vi "AlliGator Global 2-Exp + IRF Convolution Fit v2.vi"(0 "Decays":cluster{"t Array":dbl[], "Data Array":dbl[]}[](array[cluster]), 1 "Initial Parameters":dbl[](array[numeric])=[-1.0, 0.0, 0.5, 0.1, 0.5, 1.0], 2 "Optimal Offset Selection Criterion":T2, 5 "Global Fit Parameters Info":T11={"Fit Data"=variant(cluster{"t Array":dbl[], "IRF Array":dbl[]} {"t Array"=[], "IRF Array"=[]}), "Global Fit Parameter Information"={"Original Parameter Indices"=[], "# Global Parameters"=0, "# Plot Specific Parameters"=0, "Global Parameter? Array"=[]}, "# Points in Plots"=[]}, 9 "Fit Options":T14={"Show Fit Residuals"=TRUE, "Fit Model"=enum."1-Exponential", "Residual Type"=enum."Standard", "Max Decay Percentile"=0.0, "Min Decay Percentile"=0.0, "Show Full Decay"=TRUE, "Weights"=enum."Unweighted", "Fitting Method"=enum."Least Square", "Compute Parameter Uncertainties"=TRUE, "Periodic Boundaries"=TRUE, "Model Calculation"=enum."Simulation", "Period"=1.2500000000000001e-08, "Termination Criteria"={"Max Iterations"=1000, "Max Function Calls"=0, "Max Time"=1000.0, "Function Tolerance"=1e-06, "Parameter Tolerance"=1e-06, "Gradient Tolerance"=0.0, "Min Lambda"=1e-06, "Max Lambda"=1e-06, "Initial Tick Count"=0}, "Offset Resolution"=1.2500000000000001e-08, "Use Local IRF"=TRUE, "Fitting Algorithm"=enum."Levenberg-Marquardt", "Show Confidence Interval "=TRUE, "Confidence Level"=95.0} {"Confidence Level" min=0.0 max=100.0; "Offset Resolution" min=0.0; "Period" min=0.0; "Min Decay Percentile" min=0.0 max=1.0; "Max Decay Percentile" min=0.0 max=100.0}, 11 "error in (no error)":errorcluster, 12 "parameter bounds":T13, 13 "Termination Criteria":T3={"Max Iterations"=1000, "Max Function Calls"=10000, "Max Time"=1000.0, "Function Tolerance"=1e-06, "Parameter Tolerance"=1e-06, "Gradient Tolerance"=1e-06, "Min Lambda"=1e-06, "Max Lambda"=1e-06, "Initial Tick Count"=0}) -> (4 "Fit Plots Array":T1[](array[typedef]), 8 "Fit Output":T4={"best nonlinear fit"=[], "best fit parameters"=[], "R^2"=0.0, "RMSE"=0.0, "error out"={"status"=FALSE, "code"=0, "source"=""}, "Fitting Method"=enum."Least Square", "number of function calls"=0, "number of iterations"=0, "covariance"=[], "Chi 2"=0.0, "DOF"=0, "Fit Convergence Criterion"=enum."Continue", "Fitting Algorithm"=enum."Levenberg-Marquardt", "Weighted Fit"=enum."Unweighted", "Gradient"=0.0, "|Delta Chi 2|"=0.0, "|Delta Chi 2|/Chi 2"=0.0, "Max |Delta a| /|a|"=0.0, "Lambda"=-1.0, "RSS"=0.0, "AIC"=0.0, "BIC"=0.0, "Max number of function calls"=0, "Max number of iterations"=0, "IRF"={"X Array"=[], "Y Array"=[]}, "IRF Normalization Factor"=0.0, "Decay Normalization Factor"=0.0, "Number of offset fits"=0, "Weighted Chi2"=-1.0, "Unweighted Chi2"=-1.0}, 10 "Delta Best Fit Parameters":dbl[](array[numeric]), 15 "error out":errorcluster)   [LabVIEW 2021, in "AlliGator Global Decay Fit.lvlib"]
uses:
  AlliGator Global Decay Fit.lvlib
  Fits/IRF(X)PSED/Decay Fit Options v4.ctl
  Fits/Decay Convolution/Decay Model.ctl
  Fits/Residual Type.ctl
  Fits/IRF(X)PSED/Fit Weights Type v2.ctl
  Fits/Non-linear Fitting Method v2.ctl
  Fits/Fit Calculation Method.ctl
  Fits/Non-linear Fitting Algorithm.ctl
  Fits/Global Fits/Global Fit Data.ctl
  Fits/Global Fits/Global Fit Parameters Information.ctl
  Fits/Non-linear Fit Output v4.ctl
  Fits/Nonlinear Fit Method.ctl
  <vilib>/Analysis/Matrix/Datatypes/RealMatrix.ctl
  Fits/Convergence Criteria.ctl
  Graphs/XY Graph/XY Graph Plot Data.ctl
  Fits/My Fit Stopping Criteria.ctl
  Fits/Optimal Offset Selection Criterion.ctl
  Fits/Fit Plots.ctl
  Settings/AlliGator Settings List.ctl
  Fits/Decay Convolution/Fit Control Data.ctl
  Fits/Decay Convolution/Global LM model function and gradient (2-Exp + IRF) v2.vi
  Phasor/Phasor Abort Parallel Computation.vi
  Fits/Decay Convolution/Global LM model function and gradient (2-Exp, Convolved, Periodic).vi
  <vilib>/Utility/error.llb/Error Cluster From Error Code.vi
  <vilib>/ErrorRing/Error Ring.xnode
  Arrays/Arrays.lvlib
  Time/Time.lvlib
  Fits/Fits.lvlib
  Graphs/XY Graph/XY Graph Add-Ons.lvlib
  Settings/AlliGator Settings.lvlib
  Phasor/Phasor.lvlib
  Decay Fit/AlliGator Decay Fit.lvlib
  <vilib>/Analysis/Matrix/NI_Matrix.lvlib
panel:
  out "CPU (s)":dbl
  out "XY Graph":T19(graph)
  # "Offset\nBaseline\nA1\ntau1\nA2\ntau2"
  # "Offset\nBaseline\nA1\ntau 1\nA2\ntau 2"
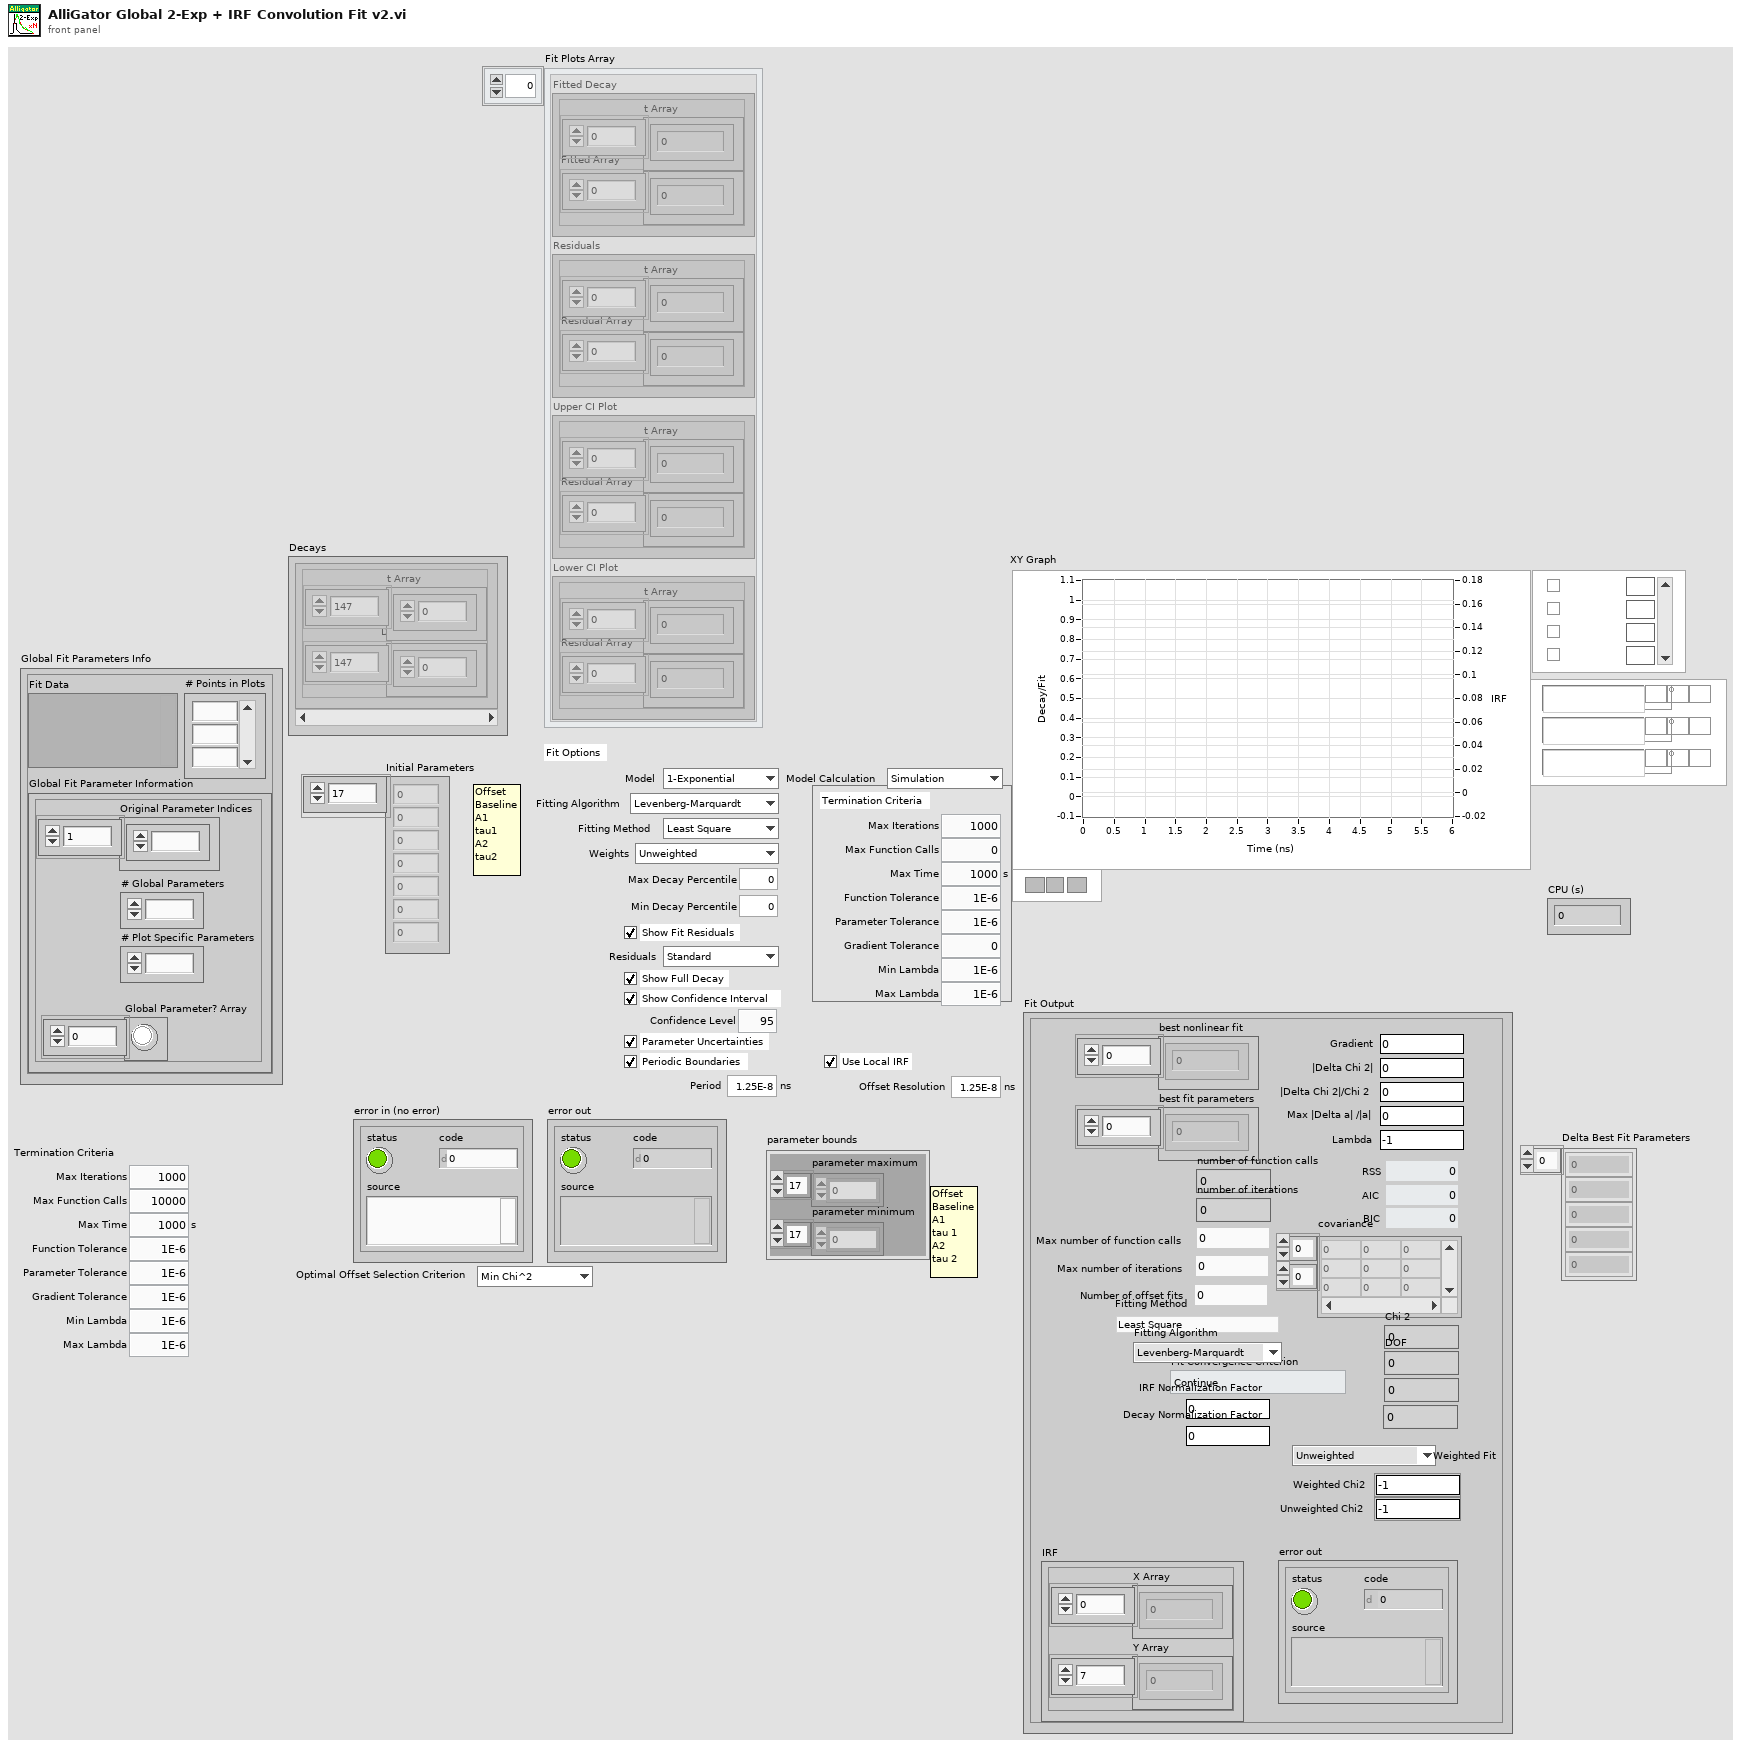
[diagram p1: front panel]
types:
  T1 = typedef "Fits.lvlib/Fit Plots.ctl" = cluster{"Fitted Decay":cluster{"t Array":dbl[], "Fitted Array":dbl[]}, "Residuals":cluster{"t Array":dbl[], "Residual Array":dbl[]}, "Upper CI Plot":cluster{"t Array":dbl[], "Residual Array":dbl[]}, "Lower CI Plot":cluster{"t Array":dbl[], "Residual Array":dbl[]}}
  T2 = typedef "Fits.lvlib/Optimal Offset Selection Criterion.ctl" = enum16{"Min Chi^2", "Max R^2"}
  T3 = typedef "Fits.lvlib/My Fit Stopping Criteria.ctl" = cluster{"Max Iterations":i32, "Max Function Calls":i32, "Max Time":dbl[unit], "Function Tolerance":dbl, "Parameter Tolerance":dbl, "Gradient Tolerance":dbl, "Min Lambda":dbl, "Max Lambda":dbl, "Initial Tick Count":u32}
  T4 = typedef "Fits.lvlib/Non-linear Fit Output v4.ctl" = cluster{"best nonlinear fit":dbl[], "best fit parameters":dbl[], "R^2":dbl, "RMSE":dbl, "error out":errorcluster, "Fitting Method":T5, "number of function calls":i32, "number of iterations":i32, "covariance":T6, "Chi 2":dbl, "DOF":i32, "Fit Convergence Criterion":T7, "Fitting Algorithm":T8, "Weighted Fit":T9, "Gradient":dbl, "|Delta Chi 2|":dbl, "|Delta Chi 2|/Chi 2":dbl, "Max |Delta a| /|a|":dbl, "Lambda":dbl, "RSS":dbl, "AIC":dbl, "BIC":dbl, "Max number of function calls":i32, "Max number of iterations":i32, "IRF":T10, "IRF Normalization Factor":dbl, "Decay Normalization Factor":dbl, "Number of offset fits":i32, "Weighted Chi2":dbl, "Unweighted Chi2":dbl}
  T5 = typedef "Fits.lvlib/Nonlinear Fit Method.ctl" = enum16{"Least Square", "Least Absolute Residual", "Bisquare", "MLE"}
  T6 = typedef "NI_Matrix.lvlib/RealMatrix.ctl" = dbl[][]
  T7 = typedef "Fits.lvlib/Convergence Criteria.ctl" = enum16{"Continue", "Tolerances Exceeded", "Max Time Exceeded", "Max Iterations Exceeded", "Max Function Evaluations Exceeded", "Scale Range Exceeded"}
  T8 = typedef "Fits.lvlib/Non-linear Fitting Algorithm.ctl" = enum16{"Levenberg-Marquardt", "Trust-Region Dogleg"}
  T9 = typedef "Fits.lvlib/Fit Weights Type v2.ctl" = enum16{"Unweighted", "1/Variance (Neyman)", "1/Variance (Pearson)", "Best of All"}
  T10 = typedef "XY Graph Add-Ons.lvlib/XY Graph Plot Data.ctl" = cluster{"X Array":dbl[], "Y Array":dbl[]}
  T11 = typedef "Fits.lvlib/Global Fit Data.ctl" = cluster{"Fit Data":variant, "Global Fit Parameter Information":T12, "# Points in Plots":i32[]}
  T12 = typedef "Fits.lvlib/Global Fit Parameters Information.ctl" = cluster{"Original Parameter Indices":i32[], "# Global Parameters":i32, "# Plot Specific Parameters":i32, "Global Parameter? Array":bool[]}
  T13 = cluster{"parameter minimum":dbl[], "parameter maximum":dbl[]}
  T14 = typedef "Fits.lvlib/Decay Fit Options v4.ctl" = cluster{"Show Fit Residuals":bool, "Fit Model":T15, "Residual Type":T16, "Max Decay Percentile":dbl, "Min Decay Percentile":dbl, "Show Full Decay":bool, "Weights":T9, "Fitting Method":T17, "Compute Parameter Uncertainties":bool, "Periodic Boundaries":bool, "Model Calculation":T18, "Period":dbl[unit], "Termination Criteria":cluster{"Max Iterations":i32, "Max Function Calls":i32, "Max Time":dbl[unit], "Function Tolerance":dbl, "Parameter Tolerance":dbl, "Gradient Tolerance":dbl, "Min Lambda":dbl, "Max Lambda":dbl, "Initial Tick Count":u32}, "Offset Resolution":dbl[unit], "Use Local IRF":bool, "Fitting Algorithm":T8, "Show Confidence Interval ":bool, "Confidence Level":dbl}
  T15 = typedef "Fits.lvlib/Decay Model.ctl" = enum16{"1-Exponential", "2-Exponentials"}
  T16 = typedef "Fits.lvlib/Residual Type.ctl" = enum16{"Standard", "Normalized", "Reduced"}
  T17 = typedef "Fits.lvlib/Non-linear Fitting Method v2.ctl" = enum16{"Least Square", "Least Absolute Residual", "Bisquare", "MLE", "-", "Best of All"}
  T18 = typedef "Fits.lvlib/Fit Calculation Method.ctl" = enum16{"Simulation", "Convolution", "Integration"}
  T19 = cluster{"t Array":dbl[], "best nonlinear fit":dbl[]}[]
  T20 = typedef "AlliGator Settings.lvlib/AlliGator Settings List.ctl" = enum16{"GUI:Visible Settings Tab", "GUI:Last Run Version", "Source Image:Use Image Histogram for Contrast", "Source Image:Low Count Pixels Rejection Options", "Source Image:High Count Pixels Rejection Options", "Source Image:Use Image Brightness", "Source Image:Blend Overlay with Image Background", "Source Image:Use Fixed ROI Diameter", "Source Image:ROI Diameter", "Source Image:ROI Center Color", "Source Image:Peak Threshold", "Source Image:Intensity Threshold", "Source Image:Image Binning Options", "Source Image:Image Smoothing Options", "Source Image:Image Histogram Active", "Source Image:Invert Binary Mask", "Source Image:Hot Pixel Removal", "Source Image:Overlay Analyzed ROI Center", "Source Image:Auto-Adjust Contrast", "Source Image:Histogram Lower Percentile", "Source Image:Histogram Upper Percentile", "Source Image:Save Source Image", "Source Image:Scale Bar Options", "Source Image:Image Resolution (Pixel Size)", "Source Image:Flatfield Correction", "Source Image:Show Dead Left Columns Correction", "Source Image:Dead Left Columns Correction", "Source Image:Image Pre-Processing Operations Order", "Source Image:Overlay ROI Median", "Source Image:Median Overlay Color", "Data Information:Gate Width", "Data Information:Nanotime Gate Separation", "Data Information:Macrotime Gate Separation", "Data Information:Gate Step", "Data Information:# Gates", "Data Information:Gate Image Exposure", "Data Information:Gate Image Integration", "Data Information:Gates to Skip", "Data Information:Gates to Keep", "Data Information:Define Gates to", "Data Information:Channel Name", "Data Information:Available Channel Names", "Data Information:Channel Arithmetic", "Data Information:Background File Subtraction", "Data Information:Background File", "Data Information:Background Scaling Factor", "Data Information:Background Pile-up Correction", "Data Information:Background Pixel Well Capacity", "Data Information:Laser Period", "Data Information:SYNC Period", "Data Information:Pile-up Correction", "Data Information:Pixel Well Capacity", "Data Information:Dataset Scaling Factor", "Fluorescence Decay_Decay Pre-Processing:Reverse Gates", "Fluorescence Decay_Decay Pre-Processing:Verbose Decay Pre-Processing", "Fluorescence Decay_Decay Pre-Processing:Use Decay Pre-Processing", "Fluorescence Decay_Decay Pre-Processing:Background Subtraction", "Fluorescence Decay_Decay Pre-Processing:Background Definition Range", "Fluorescence Decay_Decay Pre-Processing:Baseline Subtraction Method", "Fluorescence Decay_Decay Pre-Processing:Decay Pre-Processing Operations Order", "Fluorescence Decay_Decay Pre-Processing:Smoothing Parameter", "Fluorescence Decay_Decay Pre-Processing:Shift Decay", "Fluorescence Decay_Decay Pre-Processing:Decay Shift Parameters", "Fluorescence Decay_Decay Pre-Processing:Fold Decay", "Fluorescence Decay_Decay Pre-Processing:# Folds", "Fluorescence Decay_Decay Pre-Processing:1-Normalize Decay", "Fluorescence Decay_Decay Pre-Processing:[0-1]-Normalize Decay", "Fluorescence Decay_Decay Pre-Processing:Smoothen Decay", "Fluorescence Decay_Decay Pre-Processing:Extrapolate Decay", "Fluorescence Decay_Decay Pre-Processing:Use Periodicity", "Fluorescence Decay_Decay Pre-Processing:Use Cursors", "Fluorescence Decay_Decay Pre-Processing:Tail Fraction", "Fluorescence Decay_Decay Pre-Processing:Head Fraction", "Fluorescence Decay_Decay Pre-Processing:Additional Points", "Fluorescence Decay_Decay Pre-Processing:Straighten Decay", "Fluorescence Decay_Decay Pre-Processing:Constant Background", "Fluorescence Decay_Decay Pre-Processing:Pixel-Normalize Decay", "Fluorescence Decay_Advanced Analysis:Extract IRF instead of Decay", "Fluorescence Decay_Advanced Analysis:IRF Extraction Options", "Fluorescence Decay_Advanced Analysis:IRF Optimization Options", "Fluorescence Decay_Advanced Analysis:Square Pulse Options", "Fluorescence Decay_Advanced Analysis:IRF Order", "Fluorescence Decay_Advanced Analysis:IRF Time Constants", "Fluorescence Decay_Advanced Analysis:Wavelet Analysis Options", "Fluorescence Decay_Advanced Analysis:Average Lifetime Options", "Fluorescence Decay_Fit Options:Fit Options", "Fluorescence Decay_Fit Options:Use Legacy Fitting Approach", "Fluorescence Decay_Fit Options:Use Data Information Laser Period", "Fluorescence Decay_Fit Parameters:Displayed Fit Parameters", "Fluorescence Decay_Fit Parameters:Fit Parameter Constraints", "Fluorescence Decay_Fit Parameters:Export Tabulated Results", "Fluorescence Decay_Fit Parameters:MLE Baseline Offset Type", "Fluorescence Decay_Fit Parameters:MLE Baseline Offset", "Fluorescence Decay_Fit Parameters:Guess Parameter Names", "Fluorescence Decay_Fit Parameters:Guess Parameter Values", "Fluorescence Decay_Fit Parameters:Guess Parameters Options", "Fluorescence Decay_Fit Parameters:Optimal Offset Selection Criterion", "Fluorescence Decay_Styles:Show Last Decay Only", "Fluorescence Decay_Styles:Decay Graph Color Array", "Fluorescence Decay:Decay Graph Active", "Fluorescence Decay Statistics:Min Peak Value", "Fluorescence Decay Statistics:Reject Low Decay Peak Pixels", "Fluorescence Decay Statistics:Reject High Decay Peak Pixels", "Fluorescence Decay Statistics:Max Peak Value", "Time Traces:Use File Timestamp", "Time Traces:Time Step", "Time Traces:Use Intensity Correction File", "Time Traces:Intensity Correction File", "Phasor Plot:Phasor Plot Smoothing Options", "Phasor Plot:Phasor Plot Size", "Phasor Plot:Phasor Plot Graphics Options", "Phasor Plot:Cumulative Phasor Plot", "Phasor Plot:Use Phasor Brightness", "Phasor Plot:Blend Overlay with Phasor Background", "Phasor Plot:Save Phasor Plot", "Phasor Plot:Show References", "Phasor Plot:Phasor Ratio Decay Range", "Phasor Plot:Exponential Fading", "Phasor Plot:Phasor Ratio Reference Colors", "Phasor Plot:Reference Radius", "Phasor Plot:Show Color Map Vertices", "Phasor Plot:Phasor Plot Active", "Phasor Plot:Phasor Ratio Color Map Type", "Phasor Plot:Phasor Ratio Color Map", "Phasor Plot:Phasor Ratio Display Range", "Phasor Plot:Selected Image ROI(s)", "Phasor Plot:All Image ROIs", "Phasor Plot:Selected Phasor Plot ROI(s)", "Phasor Plot:All Phasor Plot ROIs", "Phasor Plot:Phasor Ratio Color-Coded Quantity", "Phasor Plot:Store Phasor Harmonics", "Phasor Plot:Draw Reference Segment", "Phasor Plot:User-Defined Quantity", "Phasor Plot:Color Scale High Color", "Phasor Plot:Color Scale Low Color", "Phasor Plot:Intensity-weighted Phasor Plot", "Phasor Graph:Phasor Frequency", "Phasor Graph:Phasor Ratio Type", "Phasor Graph:Pixel-level Phasor Computation", "Phasor Graph:Save Phasor Graph", "Phasor Graph:Phasor Graph Active", "Phasor Graph:Phasor SDV Options", "Phasor Graph:Intensity-weighted Phasor Graph", "Phasor Graph:Define Shortest Lifetime as", "Phasor Calibration:Use Backup Calibration if needed", "Phasor Calibration:Backup Calibration Type", "Phasor Calibration:Calibration Type", "Phasor Calibration:Calibration Lifetime", "Phasor Calibration:Calibration Map Algorithm", "Single-Exponential Phasor Locus (SEPL):Gate Parameters", "Single-Exponential Phasor Locus (SEPL):User-defined Gate", "Single-Exponential Phasor Locus (SEPL):User-defined IRF", "Single-Exponential Phasor Locus (SEPL):Phasor Parameters", "Single-Exponential Phasor Locus (SEPL):Decay & IRF Parameters", "Single-Exponential Phasor Locus (SEPL):Display Parameters", "Lifetime Analysis:Decay Analysis Parameters", "Lifetime Analysis:Lifetime Map Active", "Plugins:Python Settings", "Miscellaneous:Verbose Mode", "Miscellaneous:Beep after Script", "Miscellaneous:Saved Image File Format", "Miscellaneous:Exported Gate Image Settings", "Miscellaneous:Include Loading in Timing", "Miscellaneous:Verbose Settings Mode", "Miscellaneous:Histogram Options", "Miscellaneous:Beep on Error", "Miscellaneous:# Logical Processors Used", "Miscellaneous:ROI Description Max Characters", "Miscellaneous:Verbose Error Mode", "Miscellaneous:Transparent Mask Color"}
  T21 = typedef "Fits.lvlib/Fit Control Data.ctl" = cluster{"IRF":T10, "Laser Period":dbl, "SYNC Period":dbl}
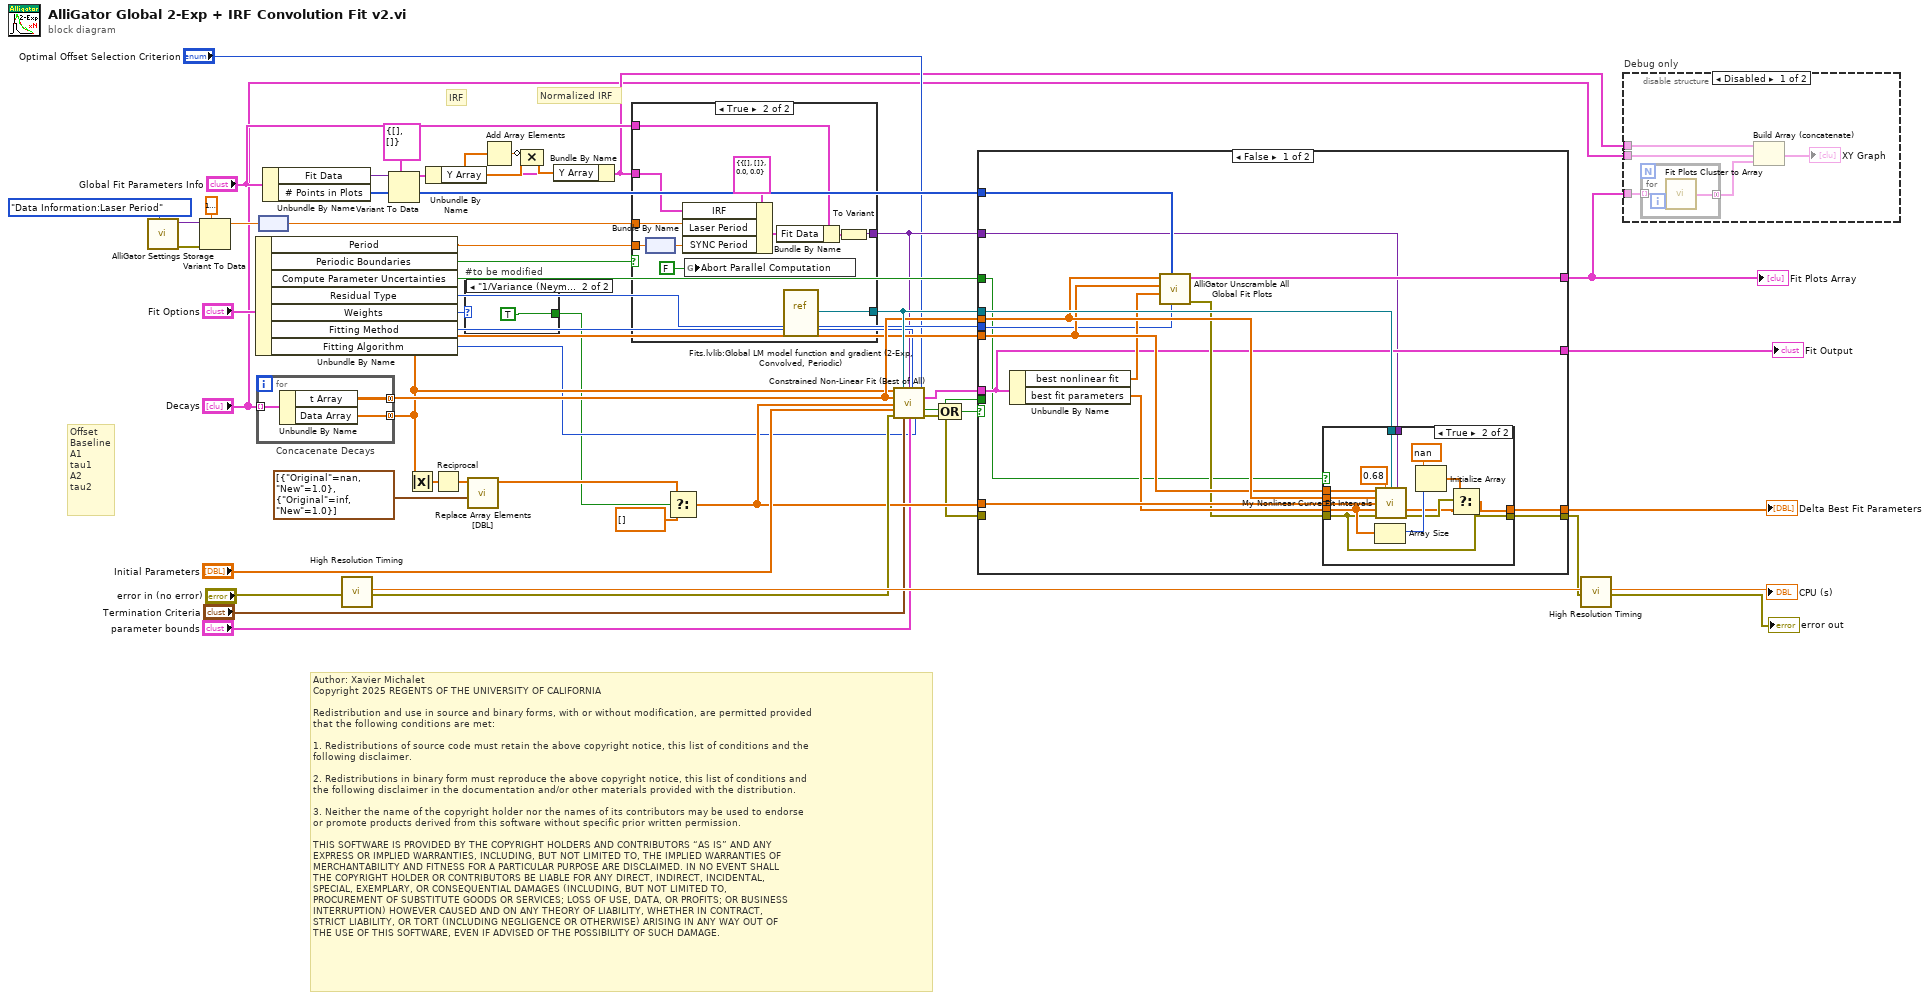
[diagram p0: block diagram]
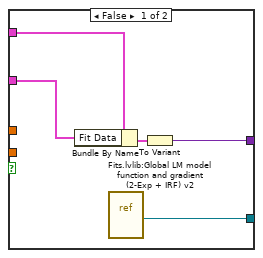
[diagram p4: hidden frame]
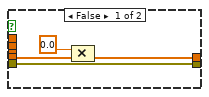
[diagram p5: hidden frame]
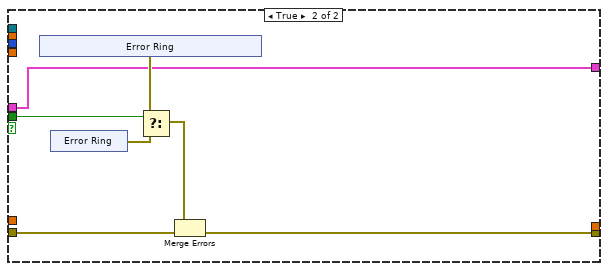
[diagram p6: hidden frame]
diagram:
  # "Author: Xavier Michalet\nCopyright 2025 REGENTS OF THE UNIVERSITY OF CALIFORNIA\n\nRedistribution and use in source and binary forms, with or without modification, are permitted provided\nthat the following conditions are met:\n\n1. Redistributions of source code must retain the above copyright notice, this list of conditions and the\nfollowing disclaimer.\n\n2. Redistributions in binary form must reproduce the above copyright notice, this list of conditions and\nthe following disclaimer in the documentation and/or other materials provided with the distribution.\n\n3. Neither the name of the copyright holder nor the names of its contributors may be used to endorse \nor promote products derived from this software without specific prior written permission.\n\nTHIS SOFTWARE IS PROVIDED BY THE COPYRIGHT HOLDERS AND CONTRIBUTORS “AS IS” AND ANY \nEXPRESS OR IMPLIED WARRANTIES, INCLUDING, BUT NOT LIMITED TO, THE IMPLIED WARRANTIES OF\nMERCHANTABILITY AND FITNESS FOR A PARTICULAR PURPOSE ARE DISCLAIMED. IN NO EVENT SHALL\nTHE COPYRIGHT HOLDER OR CONTRIBUTORS BE LIABLE FOR ANY DIRECT, INDIRECT, INCIDENTAL, \nSPECIAL, EXEMPLARY, OR CONSEQUENTIAL DAMAGES (INCLUDING, BUT NOT LIMITED TO, \nPROCUREMENT OF SUBSTITUTE GOODS OR SERVICES; LOSS OF USE, DATA, OR PROFITS; OR BUSINESS\nINTERRUPTION) HOWEVER CAUSED AND ON ANY THEORY OF LIABILITY, WHETHER IN CONTRACT, \nSTRICT LIABILITY, OR TORT (INCLUDING NEGLIGENCE OR OTHERWISE) ARISING IN ANY WAY OUT OF\nTHE USE OF THIS SOFTWARE, EVEN IF ADVISED OF THE POSSIBILITY OF SUCH DAMAGE."
  # "Normalized IRF"
  # "IRF"
  # "Offset\nBaseline\nA1\ntau1\nA2\ntau2"
  n1 = call "AlliGator Settings Storage.vi"("AlliGator Settings List"=AlliGator_Settings_List."Data Information:Laser Period") -> ("Error Out"=w16:errorcluster, "Variant Data out"=w17:variant)  [unwired: 9 in]
  n2 = Variant To Data(error in=w16, type=dbl[unit] 1e-09 ("New"), Variant=w17) -> (data=w14:dbl[unit])  [unwired: 1 out]
  n3 = Unbundle By Name("Fit Options") -> ("Period"=w9:dbl[unit], "Periodic Boundaries"=w13:bool, "Compute Parameter Uncertainties"=w21:bool, "Residual Type"=w27:T16, "Weights"=w7:T9, "Fitting Method"=w23:T17, "Fitting Algorithm"=w8:T8)
  n4 = for "Concacenate Decays" {
    tunnel: "Decays" -> [w55] mode=indexing
    tunnel: [w54] -> w29 mode=concatenating
    tunnel: [w53] -> w28 mode=concatenating
    n5 = Unbundle By Name(w55) -> ("t Array"=w54:dbl[], "Data Array"=w53:dbl[])
  }
  n6 = node(w14) -> (w10:dbl)
  n7 = Unbundle By Name("Global Fit Parameters Info") -> ("Fit Data"=w32:variant, "# Points in Plots"=w19:i32[])
  n8 = call "High Resolution Timing.vi"("Error In"="error in (no error)") -> ("elapsed (relative) seconds"=w47:dbl, "Error Out"=w38:errorcluster)  [unwired: 16 in, 1 out]
  n9 = Variant To Data(type=T10 {"X Array"=[], "Y Array"=[]} ("Plot"), Variant=w32) -> (data=w30:T10)  [unwired: 1 in, 1 out]
  n10 = Absolute Value(x=w28) -> (abs(x)=w52:dbl[])
  n11 = Unbundle By Name(w30) -> ("Y Array"=w44:dbl[])
  n12 = Reciprocal(x=w52) -> (1/x=w51:dbl[])
  n13 = case "#to be modified" shown="\"1/Variance (Neyman)\"" w7 {
    tunnel: [_ TRUE ("Weighted Fit")] -> w6
    frame "Unweighted", Default {
    }
    frame "1/Variance (Neyman)" {
    }
  }
  n14 = call "Replace Array Elements [DBL].vi"("Array of Replacement Pairs"=cluster{"Original":dbl, "New":dbl}[] [{"Original"=nan, "New"=1.0}, {"Original"=inf, "New"=1.0}], "Array"=w51) -> ("Array with Replacements"=w41:dbl[])  [unwired: 8 in, 1 out]
  n15 = Add Array Elements(numeric array=w44) -> (sum=w45:dbl)
  n16 = Compound Arithmetic op=MULTIPLY(invert w45, w44) -> (w43:dbl[])
  n17 = Bundle By Name(cluster=w30, "Y Array"=w43) -> (w3:T10)
  n18 = case shown="True" w13 {
    tunnel: [w61 w63] -> w36
    tunnel: w3 -> [w59 w71]
    tunnel: "Global Fit Parameters Info" -> [w58 w67]
    tunnel: [w57 w64] -> w11
    tunnel: w10 -> [_ w70]
    tunnel: w9 -> [_ w69]
    frame False {
      n19 = Bundle By Name(cluster=w58, "Fit Data"=w59) -> (w60:T11)
      n20 = vi-ref "Fits.lvlib:Global LM model function and gradient (2-Exp + IRF) v2.vi"() -> (w61:refnum<vi>)
      n21 = To Variant(anything=w60) -> (Variant=w57:variant)
    }
    frame True {
      n22 = node(w69) -> (w72:dbl)
      n23 = Bundle By Name(cluster=T21 {"IRF"={"X Array"=[], "Y Array"=[]}, "Laser Period"=0.0, "SYNC Period"=0.0} ("Fit Control Data"), "IRF"=w71, "Laser Period"=w70, "SYNC Period"=w72) -> (w66:T21)
      n24 = global write "Phasor Abort Parallel Computation.vi" "Abort Parallel Computation"(FALSE ("Abort Parallel Computation")) -> ()
      n25 = Bundle By Name(cluster=w67, "Fit Data"=w66) -> (w65:T11)
      n26 = vi-ref "Fits.lvlib:Global LM model function and gradient (2-Exp, Convolved, Periodic).vi"() -> (w63:refnum<vi>)
      n27 = To Variant(anything=w65) -> (Variant=w64:variant)
    }
  }
  n28 = Select(t=w41, s=w6, f=dbl[] [] ("Array with Replacements")) -> (s? t:f=w37:dbl[])
  n29 = call "Constrained Non-Linear Fit (Best of All).vi"("Y Array"=w28, "f(x,a)"=w36, "Data"=w11, "Fitting Method"=w23, "Optimal Offset Selection Criterion"="Optimal Offset Selection Criterion", "X Array"=w29, "Weights"=w37, "Guess Fitted Parameters"="Initial Parameters", "error in (no error)"=w38, "Termination Criteria"="Termination Criteria", "Fitted parameter bounds"="parameter bounds", "Fitting Algorithm"=w8) -> ("Fit Output"=w5:T4, "Fit Aborted?"=w24:bool, "Error Out"=w25:errorcluster)  [unwired: 1 out]
  n30 = Compound Arithmetic op=OR(w24, w25) -> (w26:bool)
  n31 = case shown="False" w26 {
    tunnel: [w77 _] -> w1
    tunnel: [w87 w110] -> w34
    tunnel: [w86 _] -> w35
    tunnel: w27 -> [w79 _]
    tunnel: w29 -> [w82 _]
    tunnel: w28 -> [w81 _]
    tunnel: w37 -> [w85 _]
    tunnel: w5 -> [w76 w106]
    tunnel: w36 -> [w83 _]
    tunnel: w25 -> [_ w112]
    tunnel: w24 -> [_ w111]
    tunnel: [w76 w106] -> w22
    tunnel: w21 -> [w75 _]
    tunnel: w19 -> [w74 _]
    tunnel: w11 -> [w73 _]
    frame False {
      n32 = Unbundle By Name(w76) -> ("best nonlinear fit"=w80:dbl[], "best fit parameters"=w84:dbl[])
      n33 = call "AlliGator Unscramble All Global Fit Plots.vi"("Residual Type"=w79, "# Points in Plots"=w74, "Best Nonlinear Fit Array"=w80, "Y array"=w81, "t Array"=w82) -> ("Error Out"=w78:errorcluster, "Fit Plots Array"=w77:T1[])  [unwired: 5 in]
      n34 = case shown="True" w75 {
        tunnel: w73 -> [_ w105]
        tunnel: [w91 w92] -> w87
        tunnel: [w89 w93] -> w86
        tunnel: w85 -> [_ w103]
        tunnel: w84 -> [w90 w97]
        tunnel: w83 -> [_ w102]
        tunnel: w82 -> [_ w101]
        tunnel: w81 -> [_ w100]
        tunnel: w78 -> [w91 w92]
        frame False {
          n35 = Compound Arithmetic op=MULTIPLY(0.0, w90) -> (w89:dbl[])
        }
        frame True {
          n36 = Array Size(array=w97) -> (size(s)=w98:i32)
          n37 = call "My Nonlinear Curve Fit Intervals.vi"("Y"=w100, "confidence level"=0.68, "f(x,a)"=w102, "data"=w105, "X"=w101, "Weight"=w103, "best fit parameters"=w97, "error in (no error)"=w92) -> ("delta best fit parameters"=w94:dbl[], "error out"=w96:errorcluster)  [unwired: 6 in]
          n38 = Initialize Array(nan ("element"), w98) -> (w95:dbl[])
          n39 = Select(t=w95, s=w96, f=w94) -> (s? t:f=w93:dbl[])
        }
      }
    }
    frame True {
      n40 = xnode "Error Ring"() -> ("error out"=w108:errorcluster)
      n41 = xnode "Error Ring"() -> ("error out"=w107:errorcluster)
      n42 = Select(t=w108, s=w111, f=w107) -> (s? t:f=w109:errorcluster)
      n43 = Merge Errors(w109, w112) -> (w110:errorcluster)
    }
  }
  "Delta Best Fit Parameters" <- w35
  "Fit Output" <- w22
  "Fit Plots Array" <- w1
  n44 = call "High Resolution Timing.vi"("relative seconds (NaN)"=w47, "Error In"=w34) -> ("elapsed (relative) seconds"=→"CPU (s)":dbl, "Error Out"=→"error out":errorcluster)  [unwired: 15 in, 1 out]
  n45 = disable-structure "Debug only" shown="Disabled" {
    disable-tunnel: w3 -> [w121 _]
    disable-tunnel: "Decays" -> [w120 _]
    disable-tunnel: w1 -> [w119 _]
    frame Disabled {
      n46 = for {
        tunnel: w119 -> [w123] mode=indexing
        tunnel: [w122] -> w118 mode=concatenating
        n47 = call "Fit Plots Cluster to Array.vi"("Fit Plots in"=w123) -> ("Fit Plot Array"=w122:cluster{"t Array":dbl[], "Fitted Array":dbl[]}[])
      }
      n48 = Build Array (concatenate)(w121, w118) -> ()  [unwired: 1 in, 1 out]
      "XY Graph" <- w120
    }
    frame Enabled {
    }
  }
